vi "报文解码.vi"(11 "字符串":string) -> (3 "data":T1 {"数组"."标识" items=["N"=1, "T"=2, "L"=3, "D"=4, "Z"=5, "M"=6, "hd"=7]; "数组"."污染物" items=["水温"=1, "浊度"=2, "DO"=3, "pH"=4, "ORP"=5, "比电导率"=6, "叶绿素a"=7, "氨氮"=8, "亚硝氮"=9, "硫化物"=10, "电压"=11, "温度"=12, "湿度"=13, "GPS经度"=14, "GPS纬度"=15, "BD经度"=16, "BD纬度"=17]; "数据类别" items=["水样数据"=0, "标样数据"=1, "零点核查数据"=2, "跨度核查数据"=3, "环境变量"=4, "水样数据补传"=16, "标样核查数据补传"=17, "零点核查数据补传"=18, "跨度核查数据补传"=19]})   [LabVIEW 2016, in "环境动力监测库.lvlib" / "NMEA.lvlib"]
uses:
  NMEA.lvlib
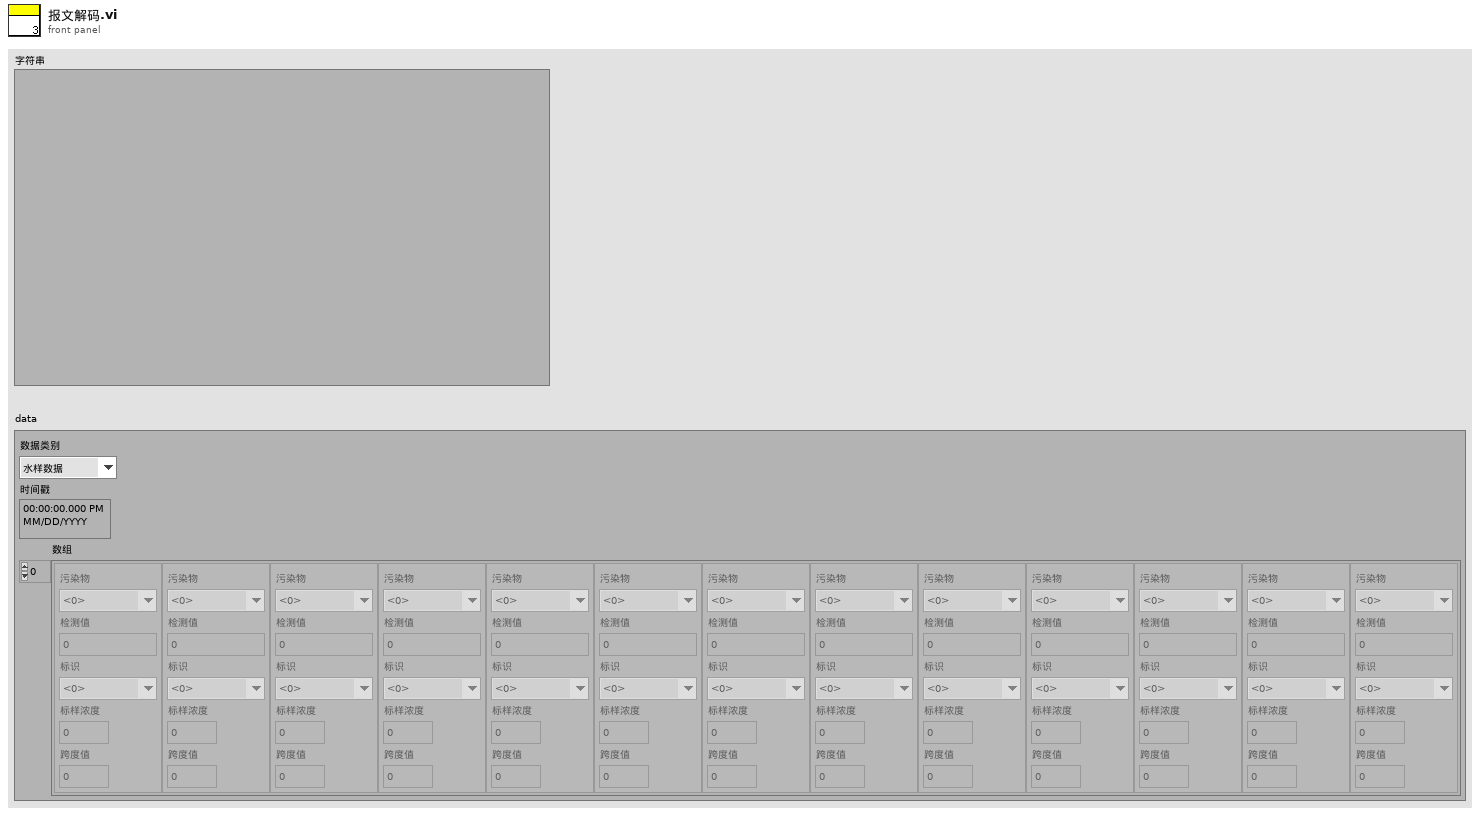
[diagram p1: front panel]
types:
  T1 = cluster{"数据类别":u16, "时间戳":timestamp, "数组":cluster{"污染物":u16, "检测值":dbl, "标识":u16, "标样浓度":dbl, "跨度值":dbl}[]}
  T2 = cluster{"污染物":u16, "检测值":dbl, "标识":u16, "标样浓度":dbl, "跨度值":dbl}
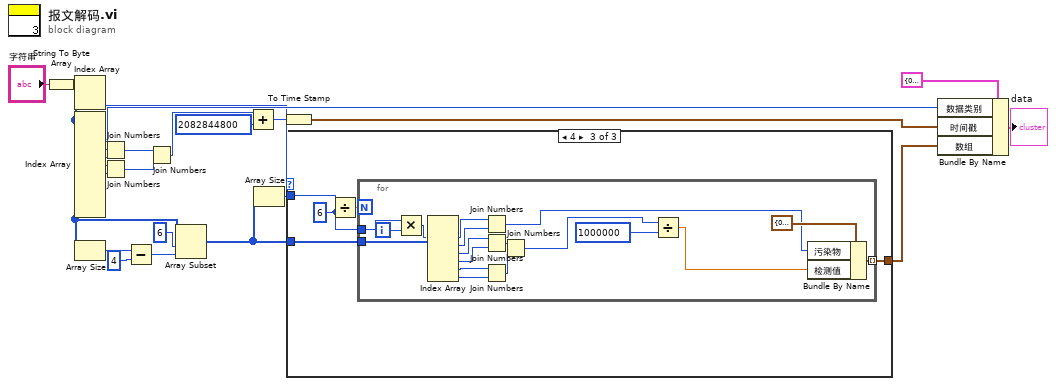
[diagram p0: block diagram]
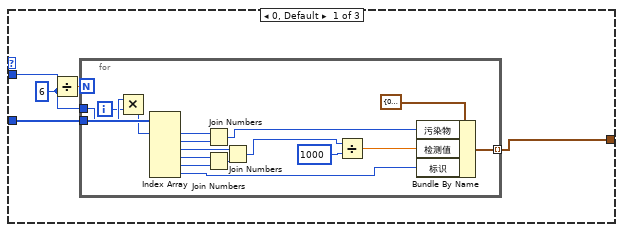
[diagram p2: hidden frame]
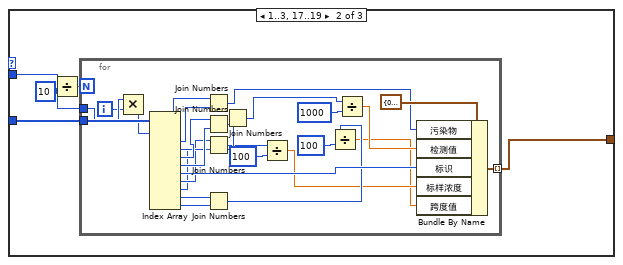
[diagram p3: hidden frame]
diagram:
  n1 = String To Byte Array(string="字符串") -> (unsigned byte array=w5:u8[])
  n2 = Index Array(array=w5) -> (element #2=w4:u8)  [unwired: 2 in, 1 out]
  n3 = Index Array(array=w5) -> (element #2=w12:u8, element #3=w22:u8, element #4=w21:u8, element #5=w20:u8, element #6=w19:u8)  [unwired: 11 in, 6 out]
  n4 = Array Size(array=w5) -> (size(s)=w9:i32)
  n5 = Join Numbers(hi=w22, lo=w21) -> ((hi.lo)=w16:u16)
  n6 = Join Numbers(hi=w20, lo=w19) -> ((hi.lo)=w17:u16)
  n7 = Subtract(x=w9, y=4) -> (x-y=w7:i32)
  n8 = Join Numbers(hi=w16, lo=w17) -> ((hi.lo)=w18:u32)
  n9 = Array Subset(array=w5, index=6 ("索引"), length=w7) -> (w3:u8[])
  n10 = Add(x=w18, y=u32 2082844800) -> (x+y=w14:u32)
  n11 = Array Size(array=w3) -> (size(s)=w2:i32)
  n12 = To Time Stamp(1:w14) -> (0:w11:timestamp)
  n13 = case shown="4" w4 {
    tunnel: w3 -> [w26 w48 w80]
    tunnel: w2 -> [w28 w50 w82]
    tunnel: [w24 w46 w78] -> w1
    frame 0, Default {
      w25 = 6 ("y")
      n14 = Divide(x=w28, y=w25) -> (x/y=w27:dbl)
      n15 = for {
        N: w27 -> [_]
        tunnel: w26 -> [w45]
        tunnel: w25 -> [w44]
        tunnel: [w38] -> w24 mode=indexing
        i -> [w43]
        n16 = Multiply(x=w44, y=w43) -> (x*y=w42:i32)
        n17 = Index Array(array=w45, index #1=w42) -> (element #1=w41:u8, element #2=w40:u8, element #3=w33:u8, element #4=w36:u8, element #5=w35:u8, element #6=w29:u8)  [unwired: 5 in]
        n18 = Join Numbers(hi=w41, lo=w40) -> ((hi.lo)=w37:u16)
        n19 = Join Numbers(hi=w36, lo=w35) -> ((hi.lo)=w34:u16)
        n20 = Join Numbers(hi=w33, lo=w34) -> ((hi.lo)=w31:u32)
        n21 = Divide(x=w31, y=u32 1000) -> (x/y=w32:dbl)
        n22 = Bundle By Name(cluster=T2 {"污染物"=0, "检测值"=0.0, "标识"=0, "标样浓度"=0.0, "跨度值"=0.0} ("数据"), "污染物"=w37, "检测值"=w32, "标识"=w29) -> (w38:T2)
      }
    }
    frame 1..3, 17..19 {
      w47 = 10 ("y")
      n23 = Divide(x=w50, y=w47) -> (x/y=w49:dbl)
      n24 = for {
        N: w49 -> [_]
        tunnel: w48 -> [w77]
        tunnel: w47 -> [w76]
        tunnel: [w70] -> w46 mode=indexing
        i -> [w75]
        n25 = Multiply(x=w76, y=w75) -> (x*y=w74:i32)
        n26 = Index Array(array=w77, index #1=w74) -> (element #1=w73:u8, element #2=w72:u8, element #3=w65:u8, element #4=w68:u8, element #5=w67:u8, element #6=w61:u8, element #7=w60:u8, element #8=w59:u8, element #9=w58:u8, element #10=w57:u8)  [unwired: 9 in]
        n27 = Join Numbers(hi=w73, lo=w72) -> ((hi.lo)=w69:u16)
        n28 = Join Numbers(hi=w68, lo=w67) -> ((hi.lo)=w66:u16)
        n29 = Join Numbers(hi=w60, lo=w59) -> ((hi.lo)=w56:u16)
        n30 = Join Numbers(hi=w58, lo=w57) -> ((hi.lo)=w55:u16)
        n31 = Join Numbers(hi=w65, lo=w66) -> ((hi.lo)=w63:u32)
        n32 = Divide(x=w56, y=u16 100) -> (x/y=w52:dbl)
        n33 = Divide(x=w55, y=u16 100) -> (x/y=w51:dbl)
        n34 = Divide(x=w63, y=u32 1000) -> (x/y=w64:dbl)
        n35 = Bundle By Name(cluster=T2 {"污染物"=0, "检测值"=0.0, "标识"=0, "标样浓度"=0.0, "跨度值"=0.0} ("数据"), "污染物"=w69, "检测值"=w64, "标识"=w61, "标样浓度"=w52, "跨度值"=w51) -> (w70:T2)
      }
    }
    frame 4 {
      w79 = 6 ("y")
      n36 = Divide(x=w82, y=w79) -> (x/y=w81:dbl)
      n37 = for {
        N: w81 -> [_]
        tunnel: w80 -> [w100]
        tunnel: w79 -> [w99]
        tunnel: [w93] -> w78 mode=indexing
        i -> [w98]
        n38 = Multiply(x=w99, y=w98) -> (x*y=w97:i32)
        n39 = Index Array(array=w100, index #1=w97) -> (element #1=w96:u8, element #2=w95:u8, element #3=w86:u8, element #4=w87:u8, element #5=w88:u8, element #6=w89:u8)  [unwired: 5 in]
        n40 = Join Numbers(hi=w96, lo=w95) -> ((hi.lo)=w92:u16)
        n41 = Join Numbers(hi=w86, lo=w87) -> ((hi.lo)=w84:u16)
        n42 = Join Numbers(hi=w88, lo=w89) -> ((hi.lo)=w85:u16)
        n43 = Join Numbers(hi=w84, lo=w85) -> ((hi.lo)=w83:u32)
        n44 = Divide(x=w83, y=u32 1000000) -> (x/y=w91:dbl)
        n45 = Bundle By Name(cluster=T2 {"污染物"=0, "检测值"=0.0, "标识"=0, "标样浓度"=0.0, "跨度值"=0.0} ("数据"), "污染物"=w92, "检测值"=w91) -> (w93:T2)
      }
    }
  }
  n46 = Bundle By Name(cluster=T1 {"数据类别"=0, "时间戳"=timestamp(0 s since 1904-01-01), "数组"=[]} ("data"), "数据类别"=w12, "时间戳"=w11, "数组"=w1) -> (→"data":T1)
